vi "Translate Protobuf Error.vi"(8 "error in":errorcluster, 10 "Error Message":string, 11 "Error Code":i32) -> (0 "error out":errorcluster)   [LabVIEW 2019, in "grpc-lvsupport.lvlib"]
uses:
  grpc-lvsupport.lvlib
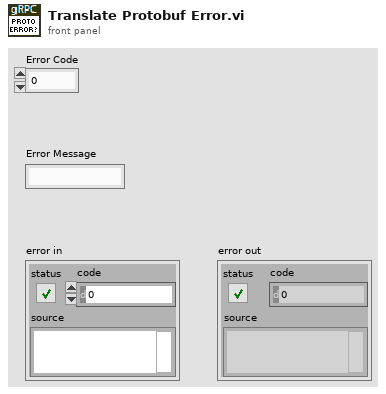
[diagram p1: front panel]
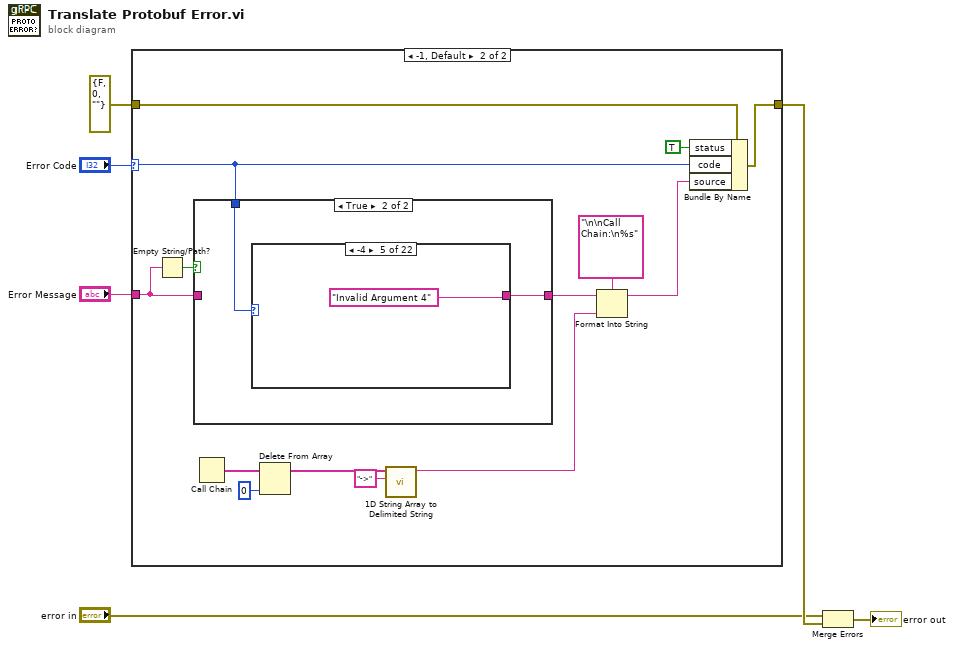
[diagram p0: block diagram]
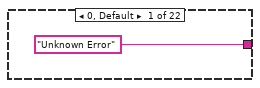
[diagram p4: hidden frame]
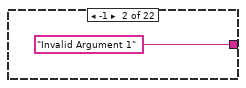
[diagram p5: hidden frame]
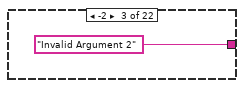
[diagram p6: hidden frame]
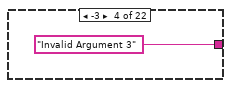
[diagram p7: hidden frame]
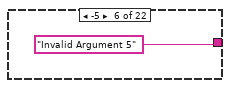
[diagram p8: hidden frame]
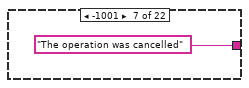
[diagram p9: hidden frame]
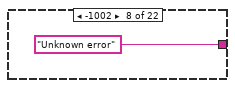
[diagram p10: hidden frame]
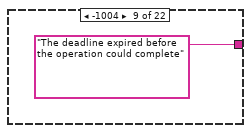
[diagram p11: hidden frame]
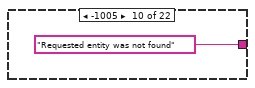
[diagram p12: hidden frame]
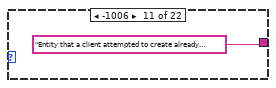
[diagram p13: hidden frame]
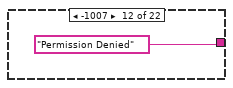
[diagram p14: hidden frame]
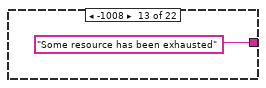
[diagram p15: hidden frame]
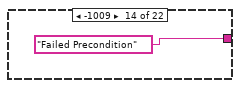
[diagram p16: hidden frame]
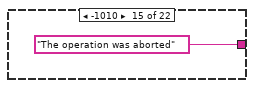
[diagram p17: hidden frame]
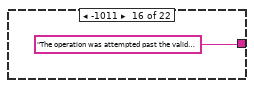
[diagram p18: hidden frame]
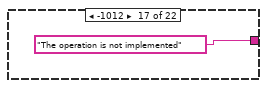
[diagram p19: hidden frame]
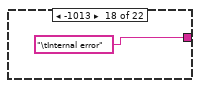
[diagram p20: hidden frame]
diagram:
  n1 = case shown="-1, Default" "Error Code" {
    selector: "Error Code" -> [_ w20]
    tunnel: [w7 w21] -> w5
    tunnel: "Error Message" -> [_ w19]
    tunnel: errorcluster {"status"=FALSE, "code"=0, "source"=""} ("error constant") -> [w7 w18]
    frame 0 {
    }
    frame -1, Default {
      n2 = Empty String/Path?(string/path=w19) -> (empty?=w16:bool)
      n3 = case shown="True" w16 {
        tunnel: w20 -> [_ w24]
        tunnel: [w22 w23] -> w15
        tunnel: w19 -> [w22 _]
        frame False {
        }
        frame True {
          n4 = case shown="-4" w24 {
            tunnel: ["Unknown Error" "Invalid Argument 1" "Invalid Argument 2" "Invalid Argument 3" "Invalid Argument 4" "Invalid Argument 5" "The operation was cancelled" "Unknown error" "The deadline expired before the operation could complete" "Requested entity was not found" "Entity that a client attempted to create already exists" "Permission Denied" "Some resource has been exhausted" "Failed Precondition" "The operation was aborted" "The operation was attempted past the valid range" "The operation is not implemented" "\tInternal error" "The service is currently unavailable" "Unrecoverable data loss or corruption" "The request does not have valid authentication credentials" "The client specified an invalid argument"] -> w23
            frame 0, Default {
            }
            frame -1 {
            }
            frame -2 {
            }
            frame -3 {
            }
            frame -4 {
            }
            frame -5 {
            }
            frame -1001 {
            }
            frame -1002 {
            }
            frame -1004 {
            }
            frame -1005 {
            }
            frame -1006 {
            }
            frame -1007 {
            }
            frame -1008 {
            }
            frame -1009 {
            }
            frame -1010 {
            }
            frame -1011 {
            }
            frame -1012 {
            }
            frame -1013 {
            }
            frame -1014 {
            }
            frame -1015 {
            }
            frame -1016 {
            }
            frame -1003 {
            }
          }
        }
      }
      n5 = Call Chain() -> (call chain=w14:string[])
      n6 = Delete From Array(array=w14, index=0) -> (array with subset deleted=w10:string[])  [unwired: 1 in, 1 out]
      n7 = call <vilib>:"1D String Array to Delimited String.vi"("delimiter"="->", "string array"=w10) -> ("delimited string"=w8:string)  [unwired: 9 in]
      n8 = Format Into String(format string="\n\nCall Chain:\n%s", initial string=w15, w8) -> (resulting string=w12:string)  [unwired: 1 in, 1 out]
      n9 = Bundle By Name(cluster=w18, "status"=TRUE, "code"=w20, "source"=w12) -> (w21:errorcluster)
    }
  }
  n10 = Merge Errors("error in", w5) -> (→"error out":errorcluster)
